vi "P2.vi"() -> ()   [LabVIEW 2021]
panel:
  in  "Boolean":bool
  out "error out 2":errorcluster
  out "String":string
  out "error out":errorcluster
  in  "Stop":bool
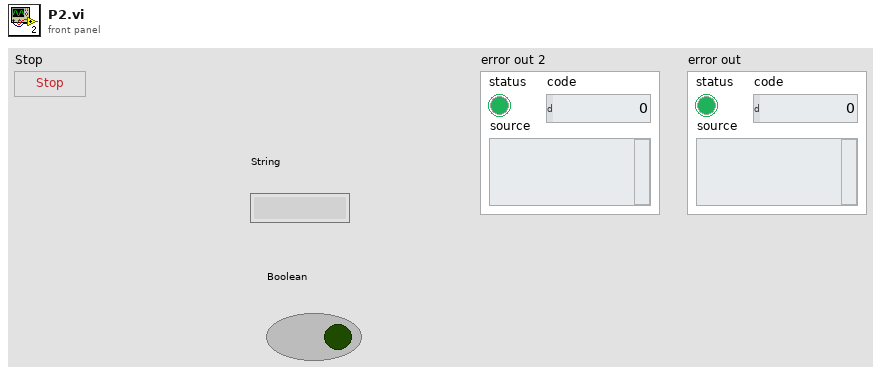
[diagram p1: front panel]
types:
  T1 = enum16{"Read", "Write", "ReadWrite", "BufferedRead", "BufferedReadWrite"}
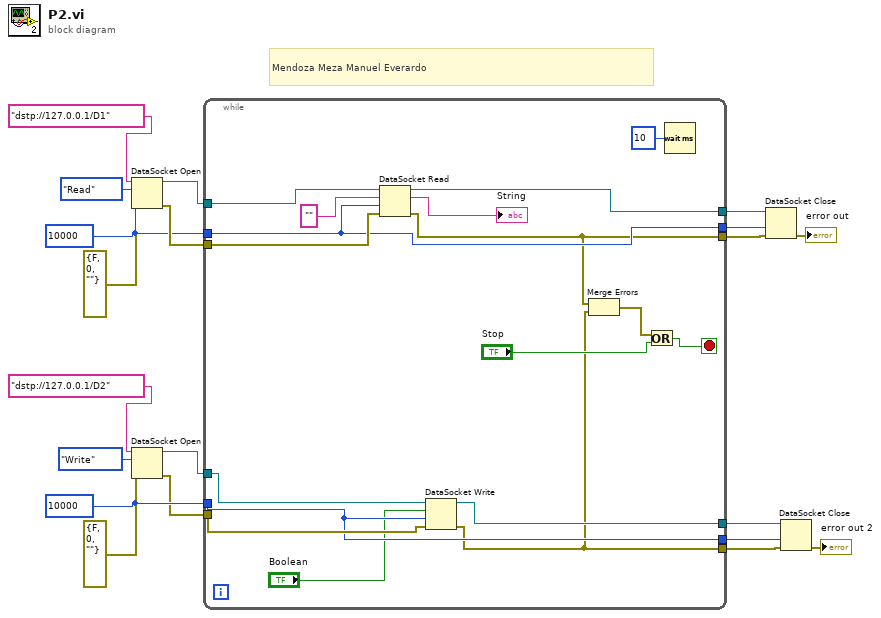
[diagram p0: block diagram]
diagram:
  w9 = 10000 ("ms timeout (10000)")
  w14 = 10000 ("ms timeout (10000)")
  # "Mendoza Meza Manuel Everardo"
  n1 = DataSocket Open(8:errorcluster {"status"=FALSE, "code"=0, "source"=""} ("error in (no error)"), 9:w14, 10:T1."Read" ("mode"), 11:"dstp://127.0.0.1/D1") -> (0:w16:errorcluster, 3:w19:refnum<k13>)
  n2 = DataSocket Open(8:errorcluster {"status"=FALSE, "code"=0, "source"=""} ("error in (no error)"), 9:w9, 10:T1."Write" ("mode"), 11:"dstp://127.0.0.1/D2") -> (0:w7:errorcluster, 3:w6:refnum<k13>)
  n3 = while {
    tunnel: w19 -> [w36]
    tunnel: [w35] -> w18
    tunnel: [w22] -> w17
    tunnel: w16 -> [w34]
    tunnel: w14 -> [w33]
    tunnel: [w33] -> w13
    tunnel: w6 -> [w27]
    tunnel: w7 -> [w30]
    tunnel: w9 -> [w29]
    tunnel: [w28] -> w1
    tunnel: [w21] -> w2
    tunnel: [w29] -> w3
    stop <- w25 stop-if-true
    n4 = DataSocket Read(8:w34, 9:w33, 10:"", 11:w36) -> (0:w22:errorcluster, 2:→"String":string, 3:w35:refnum<k13>)  [unwired: 1 in, 4 out]
    n5 = DataSocket Write(8:w30, 9:w29, 10:"Boolean", 11:w27) -> (0:w21:errorcluster, 3:w28:refnum<k13>)  [unwired: 1 out]
    n6 = Merge Errors(w22, w21) -> (w24:errorcluster)
    n7 = Or(x=w24, y="Stop") -> (x .or. y?=w25:bool)
    n8 = Wait (ms)(milliseconds to wait=u32 10) -> ()  [unwired: 1 out]
  }
  n9 = DataSocket Close(8:w17, 9:w13, 11:w18) -> (0:→"error out":errorcluster)  [unwired: 1 out]
  n10 = DataSocket Close(8:w2, 9:w3, 11:w1) -> (0:→"error out 2":errorcluster)  [unwired: 1 out]
